vi "Begin.vi"(11 "Image Size":T1=enum."160x120") -> (0 "error out":errorcluster)   [LabVIEW 2011]
doc: "Called before other user functions, this VI is expected to open initial I/O refnums, load in file data, and do all program initialization. Notice that the <B>error out</B> terminal is simply used for data flow. Wiring it to other structures or subVIs ensures that this VI runs first."
uses:
  <vilib>/Rock Robotics/WPI/Camera/WPI_CameraImageSize.ctl
  <vilib>/Rock Robotics/SystemInterfaces/Utilities/FPGA_UtilitiesLED State.ctl
  <vilib>/Rock Robotics/WPI/Joystick/WPI_JoystickDeviceEnum.ctl
  <vilib>/Rock Robotics/SystemInterfaces/DIO/FPGA_DIOChannel.ctl
  <vilib>/Rock Robotics/SystemInterfaces/AI/FPGA_AIChannel.ctl
  <vilib>/Rock Robotics/WPI/Encoder/WPI_EncoderDevRef.ctl
  <vilib>/Rock Robotics/SystemInterfaces/Encoder/FPGA_EncoderIdx.ctl
  <vilib>/Rock Robotics/SystemInterfaces/Counter/FPGA_CounterCtrSystemIndex.ctl
  <vilib>/Rock Robotics/WPI/Encoder/WPI_EncoderType.ctl
  <vilib>/Rock Robotics/WPI/AnalogChannel/WPI_AnalogChannelDevRef.ctl
  <vilib>/Rock Robotics/SystemInterfaces/Typedef/FPGA_TypedefAnalogModule.ctl
  <vilib>/Rock Robotics/WPI/MotorControl/WPI_MotorControlDeviceRef.ctl
  <vilib>/Rock Robotics/SystemInterfaces/Typedef/FPGA_TypedefDigitalModule.ctl
  <vilib>/Rock Robotics/SystemInterfaces/DIO/FPGA_DIOPWMChannel.ctl
  <vilib>/Rock Robotics/WPI/PWM/WPI_PWMDeadband.ctl
  <vilib>/Rock Robotics/WPI/CAN/Jaguar/SubVIs/WPI_CANJaguar_ControlMode.ctl
  <vilib>/Rock Robotics/WPI/PWM/WPI_PWMTransform_ConPane.ctl
  <vilib>/Rock Robotics/WPI/Relay/WPI_RelayDirection.ctl
  <vilib>/Rock Robotics/SystemInterfaces/DIO/FPGA_DIORelayChannel.ctl
  <vilib>/Rock Robotics/SystemInterfaces/Utilities/FPGA_UtilitiesLED Source.ctl
  <vilib>/Utility/file.llb/Read From Spreadsheet File (DBL).vi
  Globals/Pot Home Values.vi
  Globals/Robot Jaguars.vi
  Globals/Encoders Global.vi
  Globals/Potentiometers.vi
  Globals/Are We Calibrating Steering.vi
  Globals/Are We Calibrating Actuator.vi
  Globals/Jaguar Commands.vi
  Globals/Autonomous Joystick Emulation.vi
  Globals/Autonomous Tipping.vi
  Globals/Actuator Home Position.vi
  Globals/Max Tipper Angle.vi
  <vilib>/Rock Robotics/SystemInterfaces/AI/FPGA_AIGyroChannel.ctl
  <vilib>/Rock Robotics/WPI/Camera/WPI_CameraFrameRate.ctl
  <vilib>/Rock Robotics/WPI/Camera/WPI_CameraExposure Values.ctl
  <vilib>/Rock Robotics/WPI/Camera/WPI_CameraWhite Balance Values.ctl
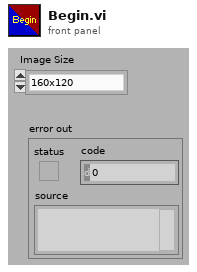
[diagram p1: front panel]
types:
  T1 = typedef "WPI_CameraImageSize.ctl" = enum16{"640x480", "320x240", "160x120"}
  T2 = typedef "FPGA_TypedefDigitalModule.ctl" = enum16{"Digital Module 1", "Digital Module 2"}
  T3 = typedef "FPGA_DIORelayChannel.ctl" = enum8{"Relay 1", "Relay 2", "Relay 3", "Relay 4", "Relay 5", "Relay 6", "Relay 7", "Relay 8", "Invalid"}
  T4 = typedef "WPI_RelayDirection.ctl" = enum16{"Both directions", "Forward only", "Reverse only"}
  T5 = typedef "FPGA_DIOChannel.ctl" = enum8{"DIO 1", "DIO 2", "DIO 3", "DIO 4", "DIO 5", "DIO 6", "DIO 7", "DIO 8", "DIO 9", "DIO 10", "DIO 11", "DIO 12", "DIO 13", "DIO 14", "Invalid"}
  T6 = typedef "FPGA_AIChannel.ctl" = enum8{"AI 1", "AI 2", "AI 3", "AI 4", "AI 5", "AI 6", "AI 7", "AI 8", "Invalid"}
  T7 = typedef "WPI_EncoderType.ctl" = enum16{"1x", "2x", "4x"}
  T8 = typedef "WPI_MotorControlDeviceRef.ctl" = cluster{"DeviceStatus":errorcluster, "Type":enum16{"PWM", "CAN"}, "PWM":cluster{"Digital Module":T2, "PWM Channel":T9, "DeadBand":T10}, "CAN":cluster{"Device Number":u8, "Control Mode":T11, "Semaphore":T12, "Max Vout":dbl}, "Invert":bool, "TransformRef":T13, "InvTransformRef":T13}
  T9 = typedef "FPGA_DIOPWMChannel.ctl" = enum8{"PWM 1", "PWM 2", "PWM 3", "PWM 4", "PWM 5", "PWM 6", "PWM 7", "PWM 8", "PWM 9", "PWM 10", "Invalid"}
  T10 = typedef "WPI_PWMDeadband.ctl" = cluster{"Name":string, "maxPositivePwm":i32, "minPositivePwm":i32, "centerPwm":i32, "maxNegativePwm":i32, "minNegativePwm":i32, "angularRange":u16}
  T11 = typedef "WPI_CANJaguar_ControlMode.ctl" = enum8{"Percent VBus", "Current", "Speed", "Position", "Voltage"}
  T12 = typedef "Semaphore RefNum" = refnum<k1>
  T13 = typedef "WPI_PWMTransform_ConPane.ctl" = refnum<vi>
  T14 = cluster{"MotorControlDevRef":T8, "MotorControlDevRef":T8, "MotorControlDevRef":T8, "MotorControlDevRef":T8, "MotorControlDevRef":T8, "MotorControlDevRef":T8, "MotorControlDevRef":T8, "MotorControlDevRef":T8}
  T15 = typedef "WPI_AnalogChannelDevRef.ctl" = cluster{"DevStatus":errorcluster, "Analog Module":T16, "Analog Channel":T6}
  T16 = typedef "FPGA_TypedefAnalogModule.ctl" = enum16{"Analog Module 1", "Analog Module 2"}
  T17 = cluster{"Front Left":T15, "Front Right":T15, "Rear Left":T15, "Rear Right":T15, "Actuator":T15}
  T18 = typedef "WPI_EncoderDevRef.ctl" = cluster{"DevStatus":errorcluster, "EncoderIndex":T19, "CounterIndex":T20, "DistancePerCount":dbl, "Decoding Type":T7}
  T19 = typedef "FPGA_EncoderIdx.ctl" = enum8{"Enc 0", "Enc 1", "Enc 2", "Enc 3", "Invalid"}
  T20 = typedef "FPGA_CounterCtrSystemIndex.ctl" = enum8{"Ctr 0", "Ctr 1", "Ctr 2", "Ctr 3", "Ctr 4", "Ctr 5", "Ctr 6", "Ctr 7", "Invalid"}
  T21 = cluster{"Front Left":T18, "Front Right":T18, "Rear Left":T18, "Rear Right":T18, "Shooter":T18}
  T22 = typedef "WPI_JoystickDeviceEnum.ctl" = enum16{"USB 1", "USB 2", "USB 3", "USB 4", "Kinect 1", "Kinect 2"}
  T23 = typedef "FPGA_UtilitiesLED State.ctl" = enum16{"Off", "On", "Toggle"}
  T24 = typedef "FPGA_UtilitiesLED Source.ctl" = enum16{"User LED", "FPGA LED"}
  T25 = typedef "WPI_JoystickDevRef.ctl" = cluster{"Device":T22}
  T26 = typedef "WPI_CameraFrameRate.ctl" = u32
  T27 = typedef "WPI_CameraExposure Values.ctl" = enum16{"Auto", "Flicker-free 50 Hz", "Flicker-free 60 Hz", "Hold current"}
  T28 = typedef "WPI_CameraWhite Balance Values.ctl" = enum16{"Auto", "Fixed indoor", "Fixed outdoor 1", "Fixed outdoor 2", "Fixed fluorescent 1", "Fixed fluorescent 2", "Hold current"}
  T29 = typedef "WPI_CameraDevRef.ctl" = cluster{"Camera Address":string, "CameraStatus":errorcluster, "Acquire Image Notifier":refnum<notifier>}
  T30 = typedef "WPI_DigitalInputDevRef.ctl" = cluster{"DevStatus":errorcluster, "DIO Channel":T5, "Digital Module":T2}
  T31 = typedef "WPI_RelayDevRef.ctl" = cluster{"DevStatus":errorcluster, "Relay Channel":T3, "Digital Module":T2, "Relay Direction":T4}
  T32 = typedef "FPGA_AIGyroChannel.ctl" = enum8{"AI 1", "AI 2", "Invalid"}
  T33 = typedef "WPI_GyroDevRef.ctl" = cluster{"DevStatus":errorcluster, "Analog Module":T16, "Analog Channel":T6, "Offset":dbl, "Gain (VoltsPerDegree/Second)":dbl}
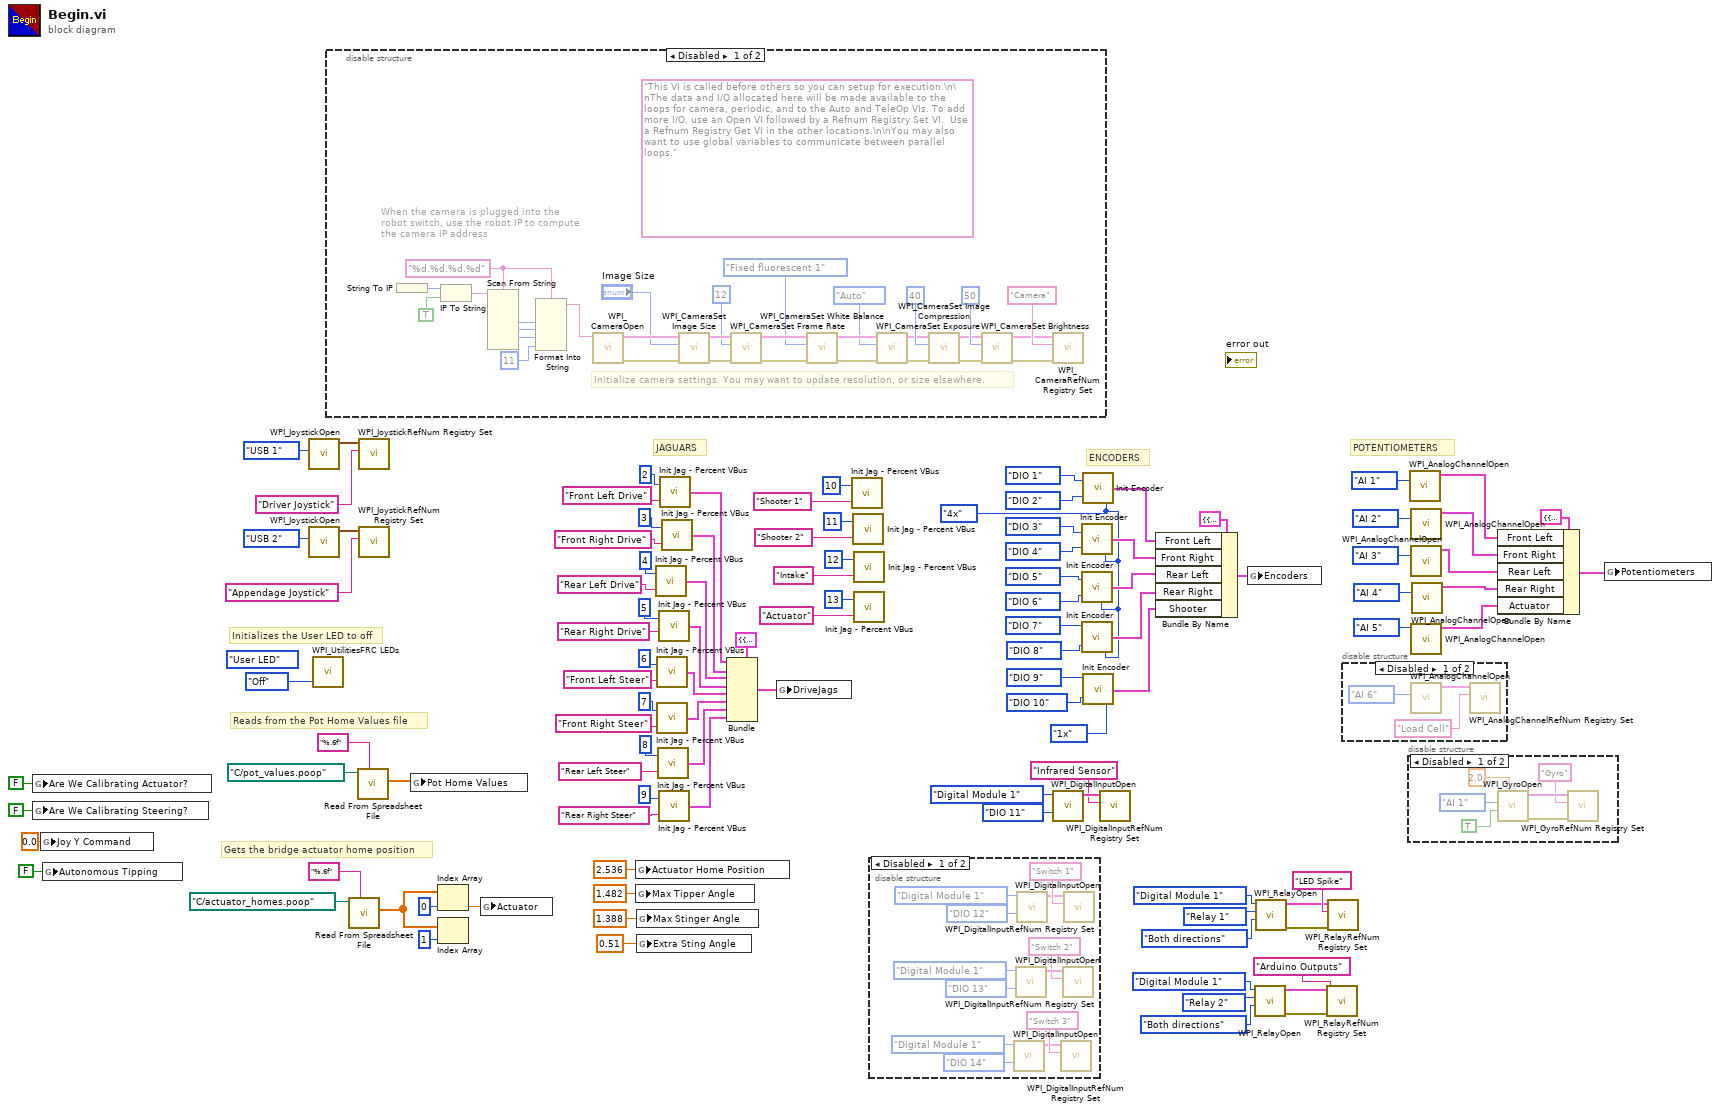
[diagram p0: block diagram]
diagram:
  w66 = WPI_EncoderType."4x" ("Decoding Type")
  (unwired) FPGA_UtilitiesLED_Source."User LED" ("LED Type")
  # "Gets the bridge actuator home position"
  # "JAGUARS"
  # "POTENTIOMETERS"
  # "ENCODERS"
  # "Reads from the Pot Home Values file"
  # "Initializes the User LED to off"
  n1 = global write "Are We Calibrating Actuator.vi" "Are We Calibrating Actuator?"(FALSE ("Are We Calibrating Actuator?")) -> ()
  n2 = global write "Are We Calibrating Steering.vi" "Are We Calibrating Steering?"(FALSE ("Are We Calibrating Steering?")) -> ()
  n3 = global write "Autonomous Joystick Emulation.vi" "Joy Y Command"(0.0 ("Joy Y Command")) -> ()
  n4 = global write "Autonomous Tipping.vi" "Autonomous Tipping"(FALSE ("Autonomous Tipping")) -> ()
  n5 = call <vilib>:"WPI_JoystickOpen.vi"("JoystickDevice"=WPI_JoystickDeviceEnum."USB 1") -> ("JoystickDevRef"=w100:T25)  [unwired: 10 in]
  n6 = call <vilib>:"WPI_JoystickOpen.vi"("JoystickDevice"=WPI_JoystickDeviceEnum."USB 2") -> ("JoystickDevRef"=w97:T25)  [unwired: 10 in]
  n7 = call <vilib>:"WPI_UtilitiesFRC LEDs.vi"("State"=FPGA_UtilitiesLED_State."Off") -> ()  [unwired: 9 in, 2 out]
  n8 = disable-structure shown="Disabled" {
    frame Disabled {
      w107 = "%d.%d.%d.%d" ("format string")
      (unwired) "This VI is called before others so you can setup for execution.\n\nThe data and I/O allocated here will be made available to the loops for camera, periodic, and to the Auto and TeleOp VIs. To add more I/O, use an Open VI followed by a Refnum Registry Set VI.  Use a Refnum Registry Get VI in the other locations.\n\nYou may also want to use global variables to communicate between parallel loops."
      # "When the camera is plugged into the\nrobot switch, use the robot IP to compute\nthe camera IP address"
      # "Initialize camera settings. You may want to update resolution, or size elsewhere."
      n9 = String To IP() -> (0:w114:u32)  [unwired: 1 in]
      n10 = IP To String(1:TRUE ("dot notation? (F)"), 2:w114) -> (0:w112:string)
      n11 = Scan From String(format string=w107, input string=w112) -> (output 1=w111:i32, output 2=w110:i32, output 3=w109:i32)  [unwired: 7 in, 3 out]
      n12 = Format Into String(format string=w107, w111, w110, w109, 11 ("Compression")) -> (resulting string=w106:string)  [unwired: 2 in, 1 out]
      n13 = call <vilib>:"WPI_CameraOpen.vi"("Camera Address"=w106) -> ("error out"=w126:errorcluster, "CameraDevRef"=w127:T29)  [unwired: 1 in, 8 out]
      n14 = call <vilib>:"WPI_CameraSet Image Size.vi"("error in (no error)"=w126, "Image Size"="Image Size", "CameraDevRef"=w127) -> ("error out"=w125:errorcluster, "CameraDevRef Out"=w128:T29)  [unwired: 7 out]
      n15 = call <vilib>:"WPI_CameraSet Frame Rate.vi"("error in (no error)"=w125, "Frame Rate (fps)"=T26 12, "CameraDevRef"=w128) -> ("error out"=w124:errorcluster, "CameraDevRef Out"=w130:T29)  [unwired: 7 out]
      n16 = call <vilib>:"WPI_CameraSet White Balance.vi"("error in (no error)"=w124, "White Balance"=WPI_CameraWhite_Balance_Values."Fixed fluorescent 1", "CameraDevRef"=w130) -> ("error out"=w123:errorcluster, "CameraDevRef Out"=w129:T29)  [unwired: 7 out]
      n17 = call <vilib>:"WPI_CameraSet Exposure.vi"("error in (no error)"=w123, "Exposure"=WPI_CameraExposure_Values."Auto", "CameraDevRef"=w129) -> ("error out"=w122:errorcluster, "CameraDevRef Out"=w132:T29)  [unwired: 7 out]
      n18 = call <vilib>:"WPI_CameraSet Image Compression.vi"("error in (no error)"=w122, "Compression"=40, "CameraDevRef"=w132) -> ("error out"=w121:errorcluster, "CameraDevRef Out"=w131:T29)  [unwired: 7 out]
      n19 = call <vilib>:"WPI_CameraSet Brightness.vi"("error in (no error)"=w121, "Brightness"=50, "CameraDevRef"=w131) -> ("error out"=w119:errorcluster, "CameraDevRef Out"=w120:T29)  [unwired: 7 out]
      n20 = call <vilib>:"WPI_CameraRefNum Registry Set.vi"("error in (no error)"=w119, "refnum name"="Camera", "CameraDevRef"=w120) -> ()  [unwired: 9 out]
    }
    frame Enabled {
    }
  }
  n21 = call-poly <vilib>:"Read From Spreadsheet File.vi"("format (%.3f)"="%.6f", "file path (dialog if empty)"=path "C:/actuator_homes.poop") -> ("first row"=w37:dbl[])  [unwired: 5 in, 4 out]
  n22 = call-poly <vilib>:"Read From Spreadsheet File.vi"("format (%.3f)"="%.6f", "file path (dialog if empty)"=path "C:/pot_values.poop") -> ("first row"=w102:dbl[])  [unwired: 5 in, 4 out]
  n23 = call <vilib>:"WPI_JoystickRefNum Registry Set.vi"("refnum name"="Driver Joystick", "JoystickDevRef"=w100) -> ()  [unwired: 8 in, 2 out]
  n24 = call <vilib>:"WPI_JoystickRefNum Registry Set.vi"("refnum name"="Appendage Joystick", "JoystickDevRef"=w97) -> ()  [unwired: 8 in, 2 out]
  n25 = global write "Pot Home Values.vi" "Pot Home Values"(w102) -> ()
  n26 = Index Array(array=w37, index=0) -> (element=w35:dbl)
  n27 = Index Array(array=w37, index=1) -> ()  [unwired: 1 out]
  n28 = global write "Jaguar Commands.vi" "Actuator"(w35) -> ()
  n29 = global write "Actuator Home Position.vi" "Actuator Home Position"(2.536 ("Actuator Home Position")) -> ()
  n30 = global write "Max Tipper Angle.vi" "Max Tipper Angle"(1.482 ("Max Tipper Angle")) -> ()
  n31 = global write "Max Tipper Angle.vi" "Max Stinger Angle"(1.388 ("Max Tipper Angle")) -> ()
  n32 = global write "Max Tipper Angle.vi" "Extra Sting Angle"(0.51 ("Max Tipper Angle")) -> ()
  n33 = call "Init Jag - Percent VBus.vi"("Jag Refnum Name"="Rear Left Drive", "Device Number"=u8 4) -> ("MotorControlDevRef"=w56:T8)
  n34 = call "Init Jag - Percent VBus.vi"("Jag Refnum Name"="Front Left Steer", "Device Number"=u8 6) -> ("MotorControlDevRef"=w17:T8)
  n35 = call "Init Jag - Percent VBus.vi"("Jag Refnum Name"="Front Right Steer", "Device Number"=u8 7) -> ("MotorControlDevRef"=w18:T8)
  n36 = call "Init Jag - Percent VBus.vi"("Jag Refnum Name"="Rear Left Steer", "Device Number"=u8 8) -> ("MotorControlDevRef"=w20:T8)
  n37 = call "Init Jag - Percent VBus.vi"("Jag Refnum Name"="Rear Right Drive", "Device Number"=u8 5) -> ("MotorControlDevRef"=w53:T8)
  n38 = call "Init Jag - Percent VBus.vi"("Jag Refnum Name"="Rear Right Steer", "Device Number"=u8 9) -> ("MotorControlDevRef"=w19:T8)
  n39 = call "Init Jag - Percent VBus.vi"("Jag Refnum Name"="Front Left Drive", "Device Number"=u8 2) -> ("MotorControlDevRef"=w64:T8)
  n40 = call "Init Jag - Percent VBus.vi"("Jag Refnum Name"="Front Right Drive", "Device Number"=u8 3) -> ("MotorControlDevRef"=w59:T8)
  n41 = Bundle(cluster=T14 {"MotorControlDevRef"={"DeviceStatus"={"status"=FALSE, "code"=0, "source"=""}, "Type"=enum."PWM", "PWM"={"Digital Module"=enum."Digital Module 1", "PWM Channel"=enum."PWM 1", "DeadBand"={"Name"="", "maxPositivePwm"=0, "minPositivePwm"=0, "centerPwm"=0, "maxNegativePwm"=0, "minNegativePwm"=0, "angularRange"=0}}, "CAN"={"Device Number"=0, "Control Mode"=enum."Percent VBus", "Semaphore"=refnum, "Max Vout"=0.0}, "Invert"=FALSE, "TransformRef"=refnum, "InvTransformRef"=refnum}, "MotorControlDevRef"={"DeviceStatus"={"status"=FALSE, "code"=0, "source"=""}, "Type"=enum."PWM", "PWM"={"Digital Module"=enum."Digital Module 1", "PWM Channel"=enum."PWM 1", "DeadBand"={"Name"="", "maxPositivePwm"=0, "minPositivePwm"=0, "centerPwm"=0, "maxNegativePwm"=0, "minNegativePwm"=0, "angularRange"=0}}, "CAN"={"Device Number"=0, "Control Mode"=enum."Percent VBus", "Semaphore"=refnum, "Max Vout"=0.0}, "Invert"=FALSE, "TransformRef"=refnum, "InvTransformRef"=refnum}, "MotorControlDevRef"={"DeviceStatus"={"status"=FALSE, "code"=0, "source"=""}, "Type"=enum."PWM", "PWM"={"Digital Module"=enum."Digital Module 1", "PWM Channel"=enum."PWM 1", "DeadBand"={"Name"="", "maxPositivePwm"=0, "minPositivePwm"=0, "centerPwm"=0, "maxNegativePwm"=0, "minNegativePwm"=0, "angularRange"=0}}, "CAN"={"Device Number"=0, "Control Mode"=enum."Percent VBus", "Semaphore"=refnum, "Max Vout"=0.0}, "Invert"=FALSE, "TransformRef"=refnum, "InvTransformRef"=refnum}, "MotorControlDevRef"={"DeviceStatus"={"status"=FALSE, "code"=0, "source"=""}, "Type"=enum."PWM", "PWM"={"Digital Module"=enum."Digital Module 1", "PWM Channel"=enum."PWM 1", "DeadBand"={"Name"="", "maxPositivePwm"=0, "minPositivePwm"=0, "centerPwm"=0, "maxNegativePwm"=0, "minNegativePwm"=0, "angularRange"=0}}, "CAN"={"Device Number"=0, "Control Mode"=enum."Percent VBus", "Semaphore"=refnum, "Max Vout"=0.0}, "Invert"=FALSE, "TransformRef"=refnum, "InvTransformRef"=refnum}, "MotorControlDevRef"={"DeviceStatus"={"status"=FALSE, "code"=0, "source"=""}, "Type"=enum."PWM", "PWM"={"Digital Module"=enum."Digital Module 1", "PWM Channel"=enum."PWM 1", "DeadBand"={"Name"="", "maxPositivePwm"=0, "minPositivePwm"=0, "centerPwm"=0, "maxNegativePwm"=0, "minNegativePwm"=0, "angularRange"=0}}, "CAN"={"Device Number"=0, "Control Mode"=enum."Percent VBus", "Semaphore"=refnum, "Max Vout"=0.0}, "Invert"=FALSE, "TransformRef"=refnum, "InvTransformRef"=refnum}, "MotorControlDevRef"={"DeviceStatus"={"status"=FALSE, "code"=0, "source"=""}, "Type"=enum."PWM", "PWM"={"Digital Module"=enum."Digital Module 1", "PWM Channel"=enum."PWM 1", "DeadBand"={"Name"="", "maxPositivePwm"=0, "minPositivePwm"=0, "centerPwm"=0, "maxNegativePwm"=0, "minNegativePwm"=0, "angularRange"=0}}, "CAN"={"Device Number"=0, "Control Mode"=enum."Percent VBus", "Semaphore"=refnum, "Max Vout"=0.0}, "Invert"=FALSE, "TransformRef"=refnum, "InvTransformRef"=refnum}, "MotorControlDevRef"={"DeviceStatus"={"status"=FALSE, "code"=0, "source"=""}, "Type"=enum."PWM", "PWM"={"Digital Module"=enum."Digital Module 1", "PWM Channel"=enum."PWM 1", "DeadBand"={"Name"="", "maxPositivePwm"=0, "minPositivePwm"=0, "centerPwm"=0, "maxNegativePwm"=0, "minNegativePwm"=0, "angularRange"=0}}, "CAN"={"Device Number"=0, "Control Mode"=enum."Percent VBus", "Semaphore"=refnum, "Max Vout"=0.0}, "Invert"=FALSE, "TransformRef"=refnum, "InvTransformRef"=refnum}, "MotorControlDevRef"={"DeviceStatus"={"status"=FALSE, "code"=0, "source"=""}, "Type"=enum."PWM", "PWM"={"Digital Module"=enum."Digital Module 1", "PWM Channel"=enum."PWM 1", "DeadBand"={"Name"="", "maxPositivePwm"=0, "minPositivePwm"=0, "centerPwm"=0, "maxNegativePwm"=0, "minNegativePwm"=0, "angularRange"=0}}, "CAN"={"Device Number"=0, "Control Mode"=enum."Percent VBus", "Semaphore"=refnum, "Max Vout"=0.0}, "Invert"=FALSE, "TransformRef"=refnum, "InvTransformRef"=refnum}}, "MotorControlDevRef"=w64, "MotorControlDevRef"=w59, "MotorControlDevRef"=w56, "MotorControlDevRef"=w53, "MotorControlDevRef"=w17, "MotorControlDevRef"=w18, "MotorControlDevRef"=w20, "MotorControlDevRef"=w19) -> (w70:T14)
  n42 = global write "Robot Jaguars.vi" "DriveJags"(w70) -> ()
  n43 = call "Init Jag - Percent VBus.vi"("Jag Refnum Name"="Shooter 1" ("refnum name"), "Device Number"=u8 10) -> ()  [unwired: 1 out]
  n44 = call "Init Jag - Percent VBus.vi"("Jag Refnum Name"="Shooter 2" ("refnum name"), "Device Number"=u8 11) -> ()  [unwired: 1 out]
  n45 = call "Init Jag - Percent VBus.vi"("Jag Refnum Name"="Intake" ("refnum name"), "Device Number"=u8 12) -> ()  [unwired: 1 out]
  n46 = call "Init Jag - Percent VBus.vi"("Jag Refnum Name"="Actuator" ("refnum name"), "Device Number"=u8 13) -> ()  [unwired: 1 out]
  n47 = disable-structure shown="Disabled" {
    frame Disabled {
      n48 = call <vilib>:"WPI_DigitalInputOpen.vi"("DIO Channel"=FPGA_DIOChannel."DIO 14", "Digital Module (Module 1)"=FPGA_TypedefDigitalModule."Digital Module 1") -> ("DigitalInputDevRef"=w136:T30)  [unwired: 8 in, 1 out]
      n49 = call <vilib>:"WPI_DigitalInputOpen.vi"("DIO Channel"=FPGA_DIOChannel."DIO 13", "Digital Module (Module 1)"=FPGA_TypedefDigitalModule."Digital Module 1") -> ("DigitalInputDevRef"=w143:T30)  [unwired: 8 in, 1 out]
      n50 = call <vilib>:"WPI_DigitalInputOpen.vi"("DIO Channel"=FPGA_DIOChannel."DIO 12", "Digital Module (Module 1)"=FPGA_TypedefDigitalModule."Digital Module 1") -> ("DigitalInputDevRef"=w144:T30)  [unwired: 8 in, 1 out]
      n51 = call <vilib>:"WPI_DigitalInputRefNum Registry Set.vi"("refnum name"="Switch 3", "DigitalInputDevRef"=w136) -> ()  [unwired: 8 in, 2 out]
      n52 = call <vilib>:"WPI_DigitalInputRefNum Registry Set.vi"("refnum name"="Switch 2", "DigitalInputDevRef"=w143) -> ()  [unwired: 8 in, 2 out]
      n53 = call <vilib>:"WPI_DigitalInputRefNum Registry Set.vi"("refnum name"="Switch 1", "DigitalInputDevRef"=w144) -> ()  [unwired: 8 in, 2 out]
    }
    frame Enabled {
    }
  }
  n54 = call <vilib>:"WPI_DigitalInputOpen.vi"("DIO Channel"=FPGA_DIOChannel."DIO 11", "Digital Module (Module 1)"=FPGA_TypedefDigitalModule."Digital Module 1") -> ("DigitalInputDevRef"=w34:T30)  [unwired: 8 in, 1 out]
  n55 = call "Init Encoder.vi"("DIO Channel A"=FPGA_DIOChannel."DIO 3", "DIO Channel B"=FPGA_DIOChannel."DIO 4", "Decoding Type"=w66) -> ("EncoderDevRef"=w77:T18)  [unwired: 1 in]
  n56 = call "Init Encoder.vi"("DIO Channel A"=FPGA_DIOChannel."DIO 5", "DIO Channel B"=FPGA_DIOChannel."DIO 6", "Decoding Type"=w66) -> ("EncoderDevRef"=w76:T18)  [unwired: 1 in]
  n57 = call "Init Encoder.vi"("DIO Channel A"=FPGA_DIOChannel."DIO 7", "DIO Channel B"=FPGA_DIOChannel."DIO 8", "Decoding Type"=w66) -> ("EncoderDevRef"=w75:T18)  [unwired: 1 in]
  n58 = call "Init Encoder.vi"("DIO Channel A"=FPGA_DIOChannel."DIO 1", "DIO Channel B"=FPGA_DIOChannel."DIO 2", "Decoding Type"=w66) -> ("EncoderDevRef"=w78:T18)  [unwired: 1 in]
  n59 = call "Init Encoder.vi"("DIO Channel A"=FPGA_DIOChannel."DIO 9", "DIO Channel B"=FPGA_DIOChannel."DIO 10", "Decoding Type"=WPI_EncoderType."1x") -> ("EncoderDevRef"=w67:T18)  [unwired: 1 in]
  n60 = call <vilib>:"WPI_DigitalInputRefNum Registry Set.vi"("refnum name"="Infrared Sensor", "DigitalInputDevRef"=w34) -> ()  [unwired: 8 in, 2 out]
  n61 = Bundle By Name(cluster=T21 {"Front Left"={"DevStatus"={"status"=FALSE, "code"=0, "source"=""}, "EncoderIndex"=enum."Invalid", "CounterIndex"=enum."Invalid", "DistancePerCount"=1.0, "Decoding Type"=enum."4x"}, "Front Right"={"DevStatus"={"status"=FALSE, "code"=0, "source"=""}, "EncoderIndex"=enum."Invalid", "CounterIndex"=enum."Invalid", "DistancePerCount"=1.0, "Decoding Type"=enum."4x"}, "Rear Left"={"DevStatus"={"status"=FALSE, "code"=0, "source"=""}, "EncoderIndex"=enum."Invalid", "CounterIndex"=enum."Invalid", "DistancePerCount"=1.0, "Decoding Type"=enum."4x"}, "Rear Right"={"DevStatus"={"status"=FALSE, "code"=0, "source"=""}, "EncoderIndex"=enum."Invalid", "CounterIndex"=enum."Invalid", "DistancePerCount"=1.0, "Decoding Type"=enum."4x"}, "Shooter"={"DevStatus"={"status"=FALSE, "code"=0, "source"=""}, "EncoderIndex"=enum."Invalid", "CounterIndex"=enum."Invalid", "DistancePerCount"=1.0, "Decoding Type"=enum."4x"}} ("Encoders"), "Front Left"=w78, "Front Right"=w77, "Rear Left"=w76, "Rear Right"=w75, "Shooter"=w67) -> (w73:T21)
  n62 = global write "Encoders Global.vi" "Encoders"(w73) -> ()
  n63 = call <vilib>:"WPI_RelayOpen.vi"("Relay Direction"=WPI_RelayDirection."Both directions", "Relay Channel"=FPGA_DIORelayChannel."Relay 2", "Digital Module (Module 1)"=FPGA_TypedefDigitalModule."Digital Module 1") -> ("error out"=w6:errorcluster, "RelayDevRef"=w1:T31)  [unwired: 7 in]
  n64 = call <vilib>:"WPI_RelayOpen.vi"("Relay Direction"=WPI_RelayDirection."Both directions", "Relay Channel"=FPGA_DIORelayChannel."Relay 1", "Digital Module (Module 1)"=FPGA_TypedefDigitalModule."Digital Module 1") -> ("error out"=w12:errorcluster, "RelayDevRef"=w7:T31)  [unwired: 7 in]
  n65 = call <vilib>:"WPI_RelayRefNum Registry Set.vi"("error in (no error)"=w6, "refnum name"="Arduino Outputs", "RelayDevRef"=w1) -> ()  [unwired: 7 in, 2 out]
  n66 = call <vilib>:"WPI_RelayRefNum Registry Set.vi"("error in (no error)"=w12, "refnum name"="LED Spike", "RelayDevRef"=w7) -> ()  [unwired: 7 in, 2 out]
  n67 = disable-structure shown="Disabled" {
    frame Disabled {
      n68 = call <vilib>:"WPI_AnalogChannelOpen.vi"("Analog Channel"=FPGA_AIChannel."AI 6") -> ("AIDeviceRef"=w149:T15)  [unwired: 9 in, 1 out]
      n69 = call <vilib>:"WPI_AnalogChannelRefNum Registry Set.vi"("refnum name"="Load Cell", "AIDeviceRef"=w149) -> ()  [unwired: 8 in, 2 out]
    }
    frame Enabled {
    }
  }
  n70 = disable-structure shown="Disabled" {
    frame Disabled {
      n71 = call <vilib>:"WPI_GyroOpen.vi"("Calibration Time (s)"=2.0, "Calibrate On Open"=TRUE, "Analog Channel"=FPGA_AIGyroChannel."AI 1") -> ("error out"=w152:errorcluster, "GyroDevRef"=w154:T33)  [unwired: 6 in, 1 out]
      n72 = call <vilib>:"WPI_GyroRefNum Registry Set.vi"("error in (no error)"=w152, "refnum name"="Gyro", "GyroDevRef"=w154) -> ()  [unwired: 7 in, 2 out]
    }
    frame Enabled {
    }
  }
  n73 = call <vilib>:"WPI_AnalogChannelOpen.vi"("Analog Channel"=FPGA_AIChannel."AI 1") -> ("AIDeviceRef"=w93:T15)  [unwired: 9 in, 1 out]
  n74 = call <vilib>:"WPI_AnalogChannelOpen.vi"("Analog Channel"=FPGA_AIChannel."AI 2") -> ("AIDeviceRef"=w89:T15)  [unwired: 9 in, 1 out]
  n75 = call <vilib>:"WPI_AnalogChannelOpen.vi"("Analog Channel"=FPGA_AIChannel."AI 3") -> ("AIDeviceRef"=w88:T15)  [unwired: 9 in, 1 out]
  n76 = call <vilib>:"WPI_AnalogChannelOpen.vi"("Analog Channel"=FPGA_AIChannel."AI 5") -> ("AIDeviceRef"=w47:T15)  [unwired: 9 in, 1 out]
  n77 = call <vilib>:"WPI_AnalogChannelOpen.vi"("Analog Channel"=FPGA_AIChannel."AI 4") -> ("AIDeviceRef"=w87:T15)  [unwired: 9 in, 1 out]
  n78 = Bundle By Name(cluster=T17 {"Front Left"={"DevStatus"={"status"=FALSE, "code"=0, "source"=""}, "Analog Module"=enum."Analog Module 1", "Analog Channel"=enum."Invalid"}, "Front Right"={"DevStatus"={"status"=FALSE, "code"=0, "source"=""}, "Analog Module"=enum."Analog Module 1", "Analog Channel"=enum."Invalid"}, "Rear Left"={"DevStatus"={"status"=FALSE, "code"=0, "source"=""}, "Analog Module"=enum."Analog Module 1", "Analog Channel"=enum."Invalid"}, "Rear Right"={"DevStatus"={"status"=FALSE, "code"=0, "source"=""}, "Analog Module"=enum."Analog Module 1", "Analog Channel"=enum."Invalid"}, "Actuator"={"DevStatus"={"status"=FALSE, "code"=0, "source"=""}, "Analog Module"=enum."Analog Module 1", "Analog Channel"=enum."Invalid"}} ("Potentiometers"), "Front Left"=w93, "Front Right"=w89, "Rear Left"=w88, "Rear Right"=w87, "Actuator"=w47) -> (w94:T17)
  n79 = global write "Potentiometers.vi" "Potentiometers"(w94) -> ()
